vi "Remove Topic Subscriber.vi"(8 "error in (no error)":errorcluster, 10 "Subscription Policy":T1, 11 "Topic in":refnum<class "Topic.lvclass">) -> (0 "error out":errorcluster, 3 "Topic out":refnum<class "Topic.lvclass">)   [LabVIEW 2015, in "Mediator.lvlib" / "Topic.lvclass"]
doc: "<License>\nCopyright © 2017 Composed Systems, LLC | All rights reserved\nwww.composed.io\n\nAuthor: Ethan Stern <ethan.stern@composed.io>\n\nThis software is provided \"AS IS\" WITHOUT WARRANTIES, either express or implied, AND IS FOR EDUCATIONAL PURPOSES ONLY.\n</License>"
uses:
  Topic.lvclass
  IMediator/ISubscriptionPolicy/ISubscriptionPolicy Reference.ctl
  IMediator/ISubscriptionPolicy/ISubscriptionPolicy.lvclass
  Topic.lvclass/Topic.ctl
  <vilib>/Utility/error.llb/Trim Whitespace.vi
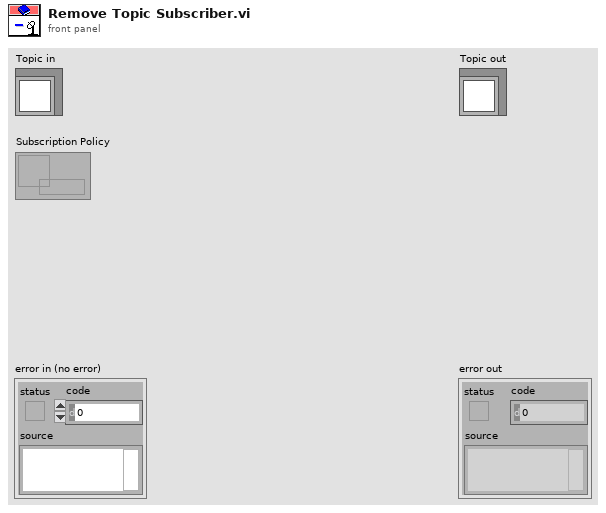
[diagram p1: front panel]
types:
  T1 = typedef "IMediator.lvlib/ISubscriptionPolicy.lvclass/ISubscriptionPolicy Reference.ctl" = refnum<data-value>
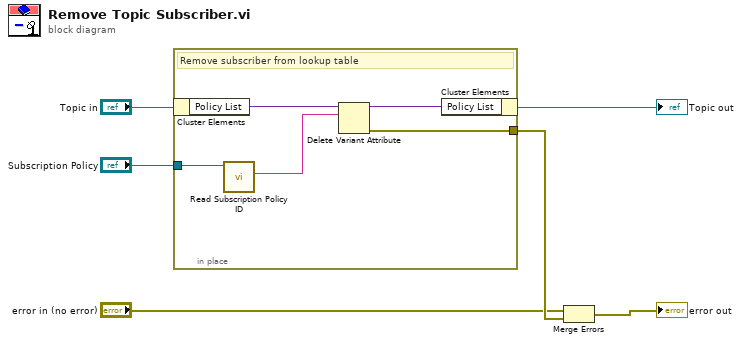
[diagram p0: block diagram]
diagram:
  n1 = in-place {
    in-place-border: [w10] -> w6
    in-place-border: "Subscription Policy" -> [w9]
    # "Remove subscriber from lookup table"
    n2 = in-place-cluster #1("Topic in") -> ("Policy List"=w8:variant)
    n3 = call "Read Subscription Policy ID.vi"("SubscriptionPolicy"=w9) -> ("Policy ID"=w7:string)  [unwired: 10 in]
    n4 = Delete Variant Attribute(6:w7, 7:w8) -> (0:w10:errorcluster, 3:w11:variant)  [unwired: 1 in, 1 out]
    n5 = in-place-cluster #1("Policy List"=w11) -> (→"Topic out":refnum<class "Topic.lvclass">)
  }
  n6 = Merge Errors("error in (no error)", w6) -> (→"error out":errorcluster)
